vi "ReadSet.vi"(3 "error in (no error)":errorcluster, 5 "VISA resource name":refnum<visa-resource-name>="COM19") -> (0 "error out":errorcluster, 1 "Set Temperature":string="set:   20.00 C\r")   [LabVIEW 2017]
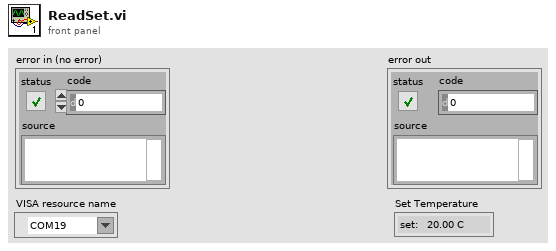
[diagram p1: front panel]
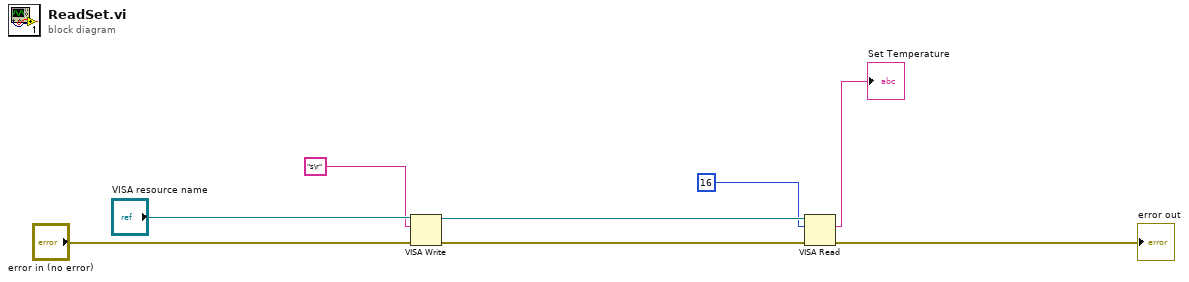
[diagram p0: block diagram]
diagram:
  n1 = VISA Write(VISA resource name="VISA resource name", write buffer="s\r", error in (no error)="error in (no error)") -> (VISA resource name out=w6:refnum<visa-resource-name>, error out=w5:errorcluster)  [unwired: 1 out]
  n2 = VISA Read(VISA resource name=w6, byte count=16, error in (no error)=w5) -> (read buffer=→"Set Temperature":string, error out=→"error out":errorcluster)  [unwired: 2 out]
